vi "LaserEnable.vi"(7 "LWSR":refnum<class "Web Request.lvclass">, 9 "Blue1":u8, 10 "Red":u8, 11 "Blue0":u8) -> ()   [LabVIEW 2014]
uses:
  <vilib>/wsapi/Web Request.lvclass
  CRDS/Actor Messages/Change Laser Enable State/Change Laser Enable State.lvclass
  Controller/Controls/Enqueuer Enum.ctl
  CRDS/Actor Messages/Change Laser Enable State/Change Laser Enable State.lvclass/Change Laser Enable State.ctl
  CRDS/Actor Messages/Change Laser Enable State/Write Blue.vi
  CRDS/Actor Messages/Change Laser Enable State/Write Red.vi
  Controller/Controller.lvclass
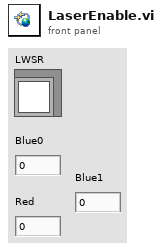
[diagram p1: front panel]
types:
  T1 = typedef "Enqueuer Enum.ctl" = enum8{"PAS", "CRDS", "File"}
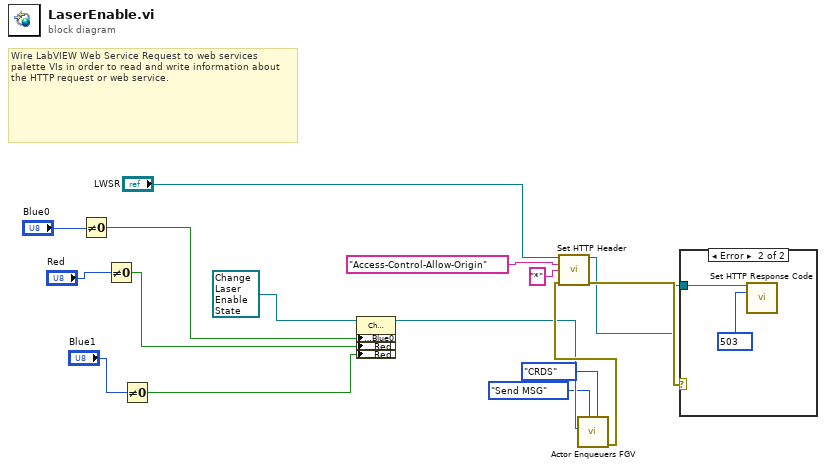
[diagram p0: block diagram]
diagram:
  # "Wire LabVIEW Web Service Request to web services palette VIs in order to read and write information about the HTTP request or web service."
  n1 = Not Equal To 0?(x="Blue0") -> (x != 0?=w7:bool)
  n2 = Not Equal To 0?(x="Red") -> (x != 0?=w6:bool)
  n3 = Not Equal To 0?(x="Blue1") -> (x != 0?=w1:bool)
  n4 = property class="Change Laser Enable State"(reference=refnum<class "Change Laser Enable State.lvclass"> refnum ("eCRDS Library.lvlib:Change Laser Enable State"), "Accessors:Blue0"=w7, "Accessors:Red"=w6, "Accessors:Red"=w1) -> (reference out=w5:refnum<class "Change Laser Enable State.lvclass">)  [unwired: 1 in, 1 out]
  n5 = call "Actor Enqueuers FGV.vi"("Enqueuer"=Enqueuer_Enum."CRDS", "State"=enum16{"Store", "Send MSG"}."Send MSG", "MSG"=w5) -> ("error out"=w11:errorcluster)  [unwired: 8 in]
  n6 = call <vilib>:"Set HTTP Header.vi"("LabVIEW Web Service Request"="LWSR", "header"="Access-Control-Allow-Origin", "header value"="*", "error in (no error)"=w11) -> ("LabVIEW Web Service Request out"=w12:refnum<class "Web Request.lvclass">, "error out"=w13:errorcluster)  [unwired: 10 in]
  n7 = case shown="Error" w13 {
    tunnel: w12 -> [_ w18]
    frame No Error {
    }
    frame Error {
      w17 = 503 items=["100"=100, "101"=101, "200"=200, "201"=201, "202"=202, "203"=203, "204"=204, "205"=205, "206"=206, "300"=300, "301"=301, "302"=302, "303"=303, "304"=304, "305"=305, "306"=306, "307"=307, "400"=400, "401"=401, "402"=402, "403"=403, "404"=404, "405"=405, "406"=406, "407"=407, "408"=408, "409"=409, "410"=410, "411"=411, "412"=412, "413"=413, "414"=414, "415"=415, "416"=416, "417"=417, "500"=500, "501"=501, "502"=502, "503"=503, "504"=504, "505"=505] ("response code (200)")
      n8 = call <vilib>:"Set HTTP Response Code.vi"("LabVIEW Web Service Request"=w18, "response code (200)"=w17) -> ()  [unwired: 12 in, 2 out]
    }
  }
